vi "SNR_Analysis.vi"(5 "Ain (Input)":ext[](array[numeric])=array[16384 elements] format="%.2f", 7 "Input Ain Freq. (Hz)":dbl=10.0 format="%.4f", 8 "AC Analysis Parameters":T1={"DC Leakage"=5, "Number of Harmonics"=6, "HarmLeakage"=3, "FundLeakage"=15, "LoFreq (Hz)"=50.0, "HiFreq (Hz)"=100.0, "Window"=enum."None ", "Reference"=TRUE} {"HiFreq (Hz)" format="%.3g"; "LoFreq (Hz)" format="%.3g"; "FundLeakage" min=1 step=2; "HarmLeakage" min=1 step=2; "DC Leakage" min=1 step=1}, 9 "Ideal Sampling Rate":dbl=500.0 format="%.4f", 10 "Number of Bits":i8=24, 11 "Number of Samples":i32=16384) -> (0 "PSRR/CMRR/BW":T2={"Freq (Hz)"=[[0.0, 49.98779296875], [49.98779296875, 100.006103515625], [100.006103515625, 149.993896484375], [149.993896484375, 200.01220703125], [200.01220703125, 250.0], [0.0, 250.0], [49.98779296875, 100.006103515625]], "SNR (dBFS)"=[122.49294424672361, 122.35389846356063, 122.34393026582947, 122.45111299294416, 122.45121773152403, 115.43161378863995, 122.35389846356063], "Fund(dB)"=0.0} {"SNR (dBFS)" format="%.2f"; "Freq (Hz)" format="%.2f"}, 1 "FFT Magnitude Plot (dB)":cluster{i32, dbl, dbl[]}(graph)={0, 0.030517578125, array[8193 elements]}, 3 "ACParameter":T3)   [LabVIEW 2010]
uses:
  Controls/TYP_ACAnalysisParam.ctl
  <vilib>/Analysis/0measdsp.llb/Scaled Time Domain Window (DBL).vi
  <vilib>/Analysis/2dsp.llb/Real FFT.vi
  <vilib>/Analysis/4window.llb/General Cosine Window (DBL).vi
  <vilib>/Analysis/NI_AALPro.lvlib
  <vilib>/Analysis/NI_AALBase.lvlib
panel:
  in  "Case Constant\n(See Context Help) 2":bool=TRUE
  in  "Case Constant\n(See Context Help)":bool
  out "Fund (compensated)":ext=17592184028025.883722 format="%.2f"
  out "Freq (Hz)":dbl[][](array[numeric])=[[0.0, 49.98779296875], [49.98779296875, 100.006103515625], [100.006103515625, 149.993896484375], [149.993896484375, 200.01220703125], [200.01220703125, 250.0], [0.0, 250.0], [49.98779296875, 100.006103515625]] format="%.2f"
  out "SNR (dBFS)":dbl[](array[numeric])=[122.49294424672361, 122.35389846356063, 122.34393026582947, 122.45111299294416, 122.45121773152403, 115.43161378863995, 122.35389846356063] format="%.2f"
  out "CoherentGain":dbl=1.0
  out "EBW":dbl=1.0
  out "Window comp (dB)":dbl=-1.9937488104915246e-08
  out "Captured Data In Plot":ext[](graph)
  out "0dB Ref (Vrms^2)":ext=17592183947264.086
  out "0dB Ref (dB)":dbl=132.45319757443235
  out "Amplitude":dbl=8388607.5
  in  "BandMultiplier":ext=1.0 format="%#.2g"
  out "Noise Floor":ext[](array[numeric])=[9.9088974720743699205, 10.2312786546159955785, 10.254789094296063996, 10.0048011243385777027, 10.004559841966981927, 50.368426126531911098, 10.2312786546159955785] format="%_2f"
  out "Power Spec\n(No DC, Fund, Harmonics)":ext[](array[numeric]) format="%.2f"
  out "Numeric":i32=16
  out "Fund(dB)":dbl=132.45319759436984 format="%.2f"
  out "SNR 2":dbl=115.43161378863995 caption="SNR (dBFS)" format="%.2f"
  out "THD (dBc)":dbl=142.87642226580417 format="%.2f"
  out "Sum of Harms 2":ext=0.090714671632502579776 format="%.2f"
  out "SF":ext=132.453188236702958824 format="%.2f"
  out "WoSpur (dBFS)":ext=-145.06459832693680674 format="%.2f"
  out "Sum of Noise 2":ext=50.368426126531911098 format="%.2f"
  out "# of Harmonics (SNR)":u32=23
  out "debug waveform":ext[](graph)
  out "FFT":dbl[](graph)
  in  "Calculate (Actual)":bool
  out "Actual Ain Freq. (Hz)":ext=10.040283203125 format="%.6f"
  out "Low Code":i32=8388619
  out "High Code":i32=-8388612
  out "Performance Array":dbl[](array[numeric])=[115.43161378863995, 145.97359756076744, 154.47799816290882, 151.76114324149736, 115.39522693755671, 142.87642226580417, 148.72341540579788, 152.36692825715133, 18.876283544444636, 18.8823278718671, 8.453417793882701e-06] format="%.2f"
  out "Ampl.":dbl=8.453417793882701e-06 format="%.2f"
  out "3rdHarm@ Plot (dB)":dbl=-152.98466091578587 format="%.2f"
  out "2ndHarm @ Plot (dB)":dbl=-168.88785823900827 format="%.2f"
  out "1stHarm @ Plot (dB)":dbl=1.9937459683205816e-08 format="%.2f"
  out "5th HD":dbl=152.36692825715133 format="%.2f"
  out "4th HD":dbl=148.72341540579788 format="%.2f"
  out "Actual Sampling Rate":dbl=500.0 format="%.6f"
  out "Measured % of FS":dbl=100.00009732361634 format="%.2f"
  out "Actual Number of Codes":u32=16777216
  out "min Code":i32
  out "max Code":i32=16777215
  out "enob":dbl=18.8823278718671 format="%.2f"
  out "ENOB":dbl=18.876283544444636 format="%.2f"
  out "3rd HD":dbl=151.76114324149736 format="%.2f"
  out "2nd HD (dBc)":dbl=154.47799816290882 format="%.2f"
  out "SFDR (dBc)":dbl=145.97359756076744 format="%.2f"
  out "THD (dBc)":dbl=136.05208345742915 format="%.2f"
  out "SNR":dbl=115.43272182505751 caption="SNR (dBc)" format="%.2f"
  out "SNRD":dbl=115.39522693755671 caption="SNRD (dBFS)" format="%.2f"
  out "max Harmonic":ext=0.044459032074172995111 format="%.2f"
  out "Fund":ext=17592184028025.883722 format="%.2f"
  out "Harmonic Spectrum":ext[](array[numeric])=[0.006273645043968196789, 0.011727499829014819744, 0.023603598512384399172, 0.010200628560604323592, 0.010739693568795177, 0.028169606117735663479, 0.022250863209773356736, 0.024737167818243943097, 0.029718462590962836569, 0.018866757624148633877, 0.01857286143792718754, 0.012624382823140385245, 0.0088173049746291707555, 0.0150888701235834066326, 0.03351059535541610953, 0.010733796961532902247, 0.044459032074172995111, 0.024528219551121035937, 0.005135965514516267305, 0.0023413793635542205077, 0.012309499745878399, 0.041509770726511618748, 0.020708228636082309619] format="%.2f"
  out "Sum of Noise":ext=50.355577026708861234 format="%.2f"
  out "Sum of Harms":ext=0.436627830163697358 format="%.2f"
  out "Bin Locations":i32[](array[numeric])
  out "Tone Bin#":u32=329
  out "Nyquist":i32=8192
  out "FFT Power Spectrum":ext[](array[numeric]) format="%.2f"
  out "Amplitude Compensation":ext=0.9999980535305147 format="%.6f"
  out "Half of Codes":ext=8388608.0 format="%.2f"
  out "Ain":ext[](array[numeric]) format="%.2f"
  # "AC Analysis"
  # "Fs"
  # "Fin"
  # "dBFS"
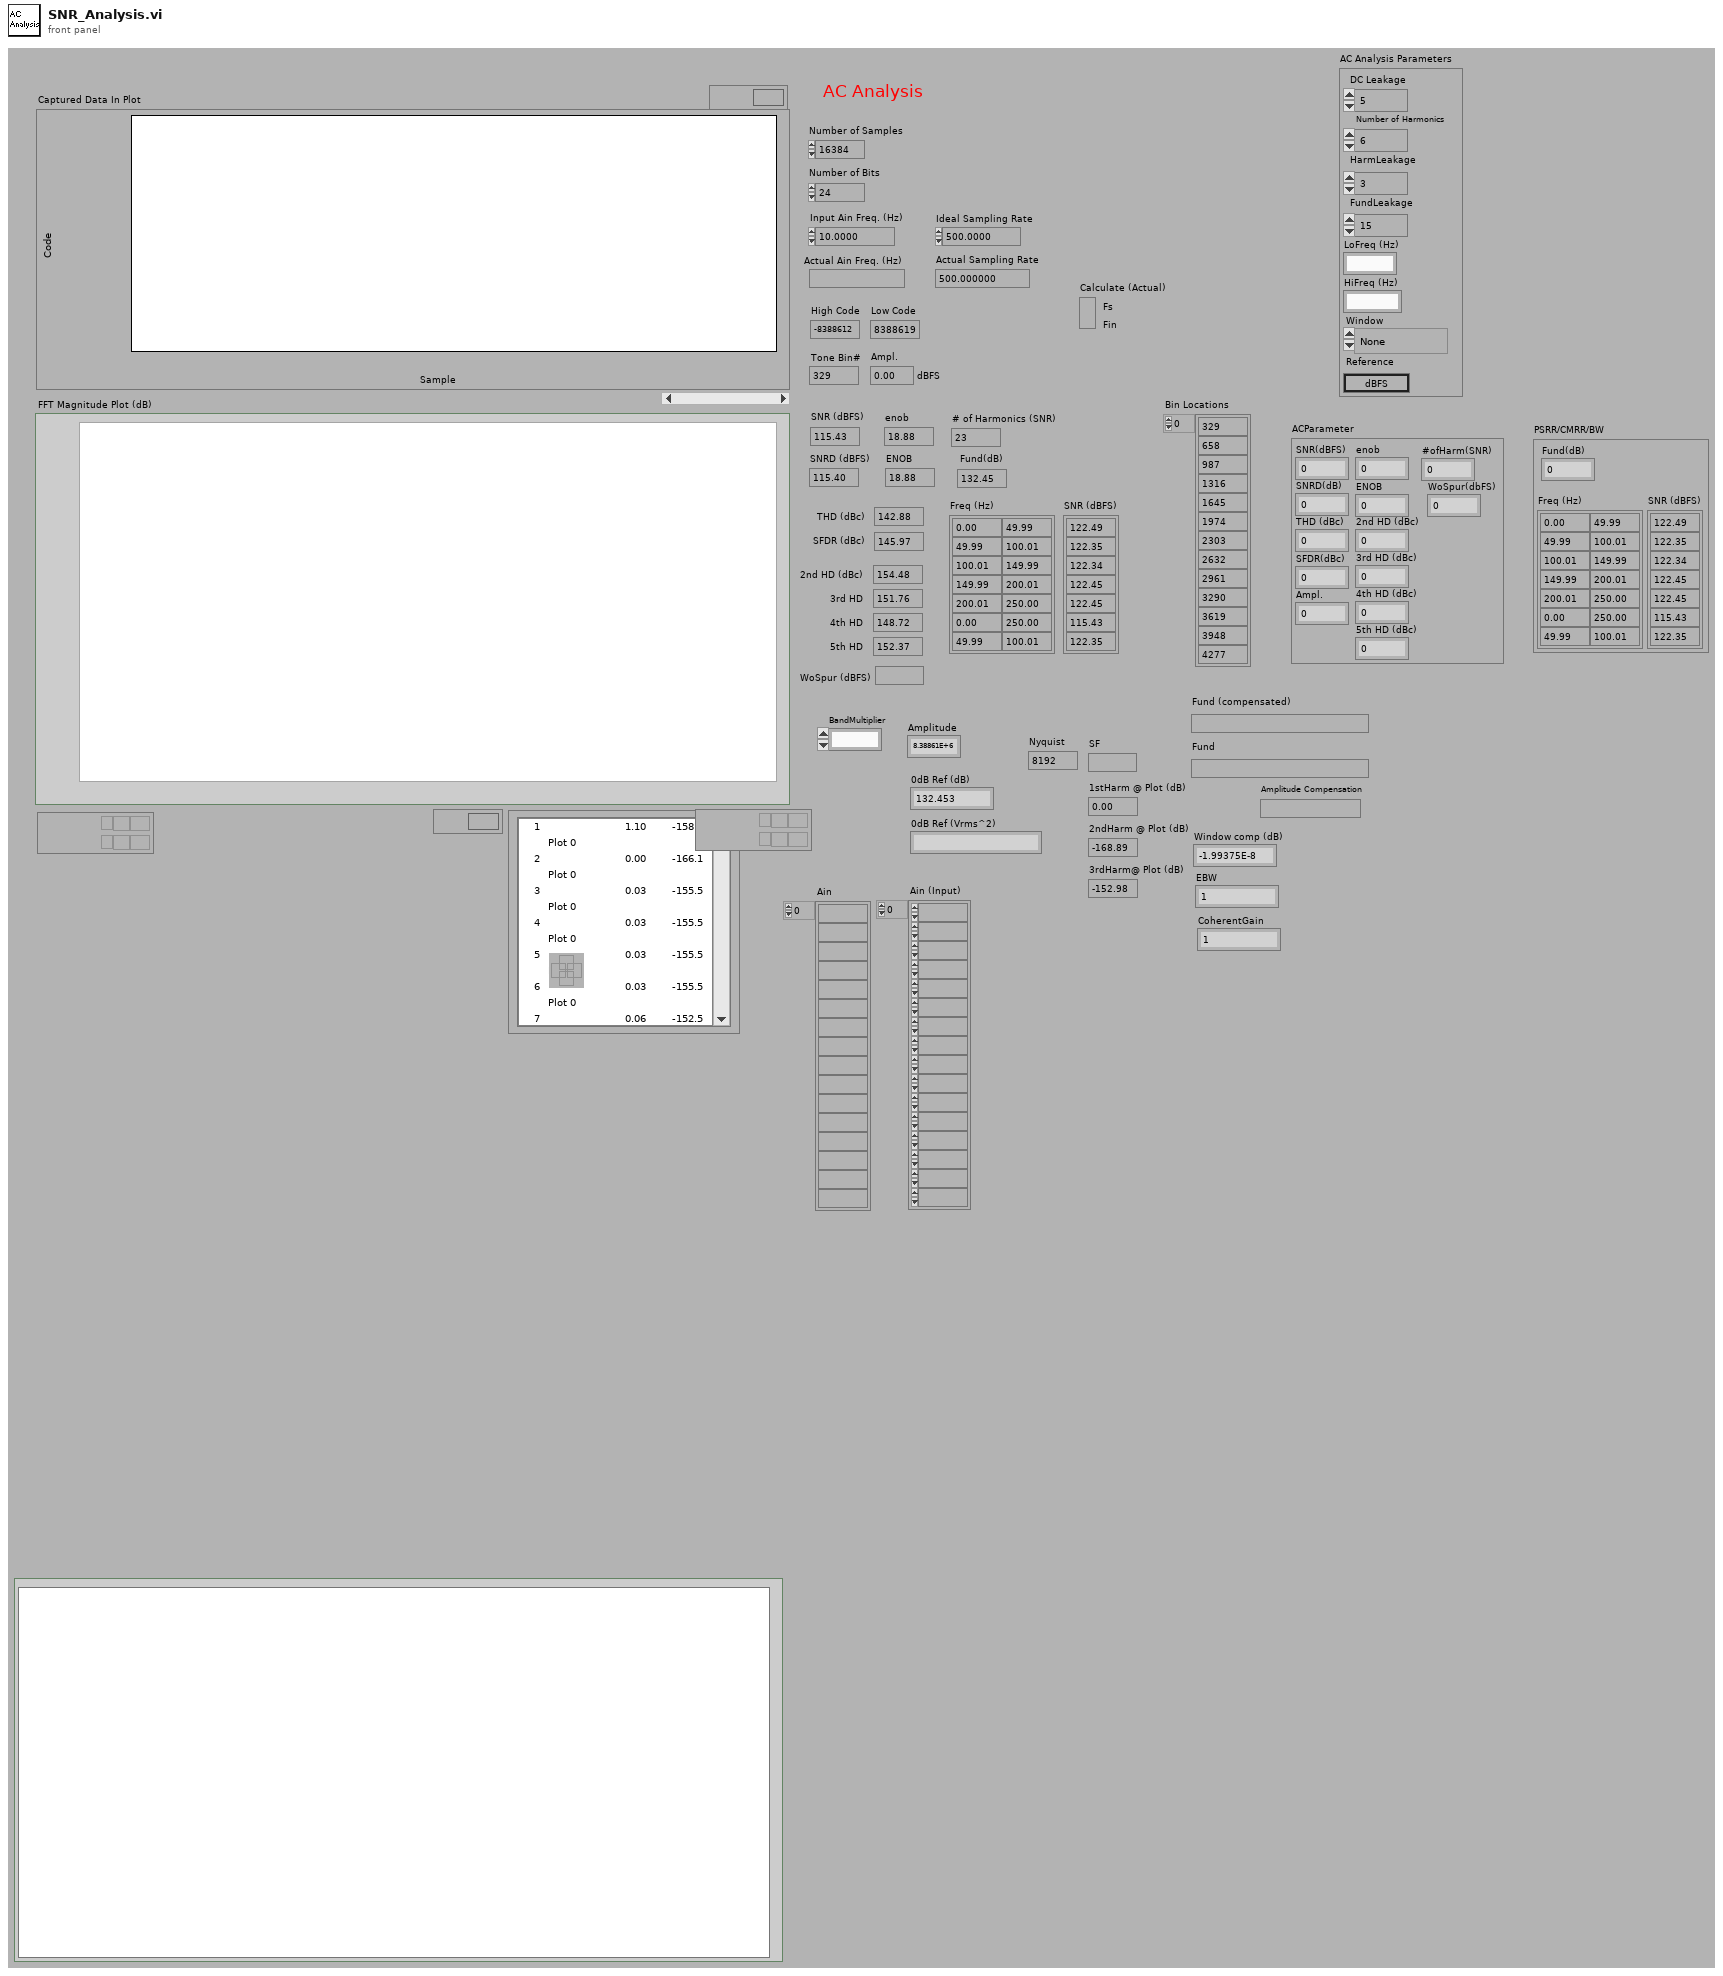
[diagram p1: front panel]
types:
  T1 = typedef "TYP_ACAnalysisParam.ctl" = cluster{"DC Leakage":i8, "Number of Harmonics":i8, "HarmLeakage":i8, "FundLeakage":i32, "LoFreq (Hz)":ext, "HiFreq (Hz)":ext, "Window":enum16{"None ", "Hanning", "Hamming", "Blackman-Harris", "Exact Blackman", "Blackman", "Flat Top", "4 Term B-Harris ", "7 Term B-Harris", "Low Sidelobe"}, "Reference":bool}
  T2 = cluster{"Freq (Hz)":dbl[][], "SNR (dBFS)":dbl[], "Fund(dB)":dbl}
  T3 = cluster{"SNR(dBFS)":dbl, "SNRD(dB)":dbl, "THD (dBc)":dbl, "SFDR(dBc)":dbl, "ENOB":dbl, "enob":dbl, "#ofHarm(SNR)":dbl, "WoSpur(dbFS)":dbl, "2nd HD (dBc)":dbl, "3rd HD (dBc)":dbl, "4th HD (dBc)":dbl, "5th HD (dBc)":dbl, "Ampl.":dbl}
  T4 = enum16{"None ", "Hanning", "Hamming", "Blackman-Harris", "Exact Blackman", "Blackman", "Flat Top", "4 Term B-Harris ", "7 Term B-Harris", "Low Sidelobe"}
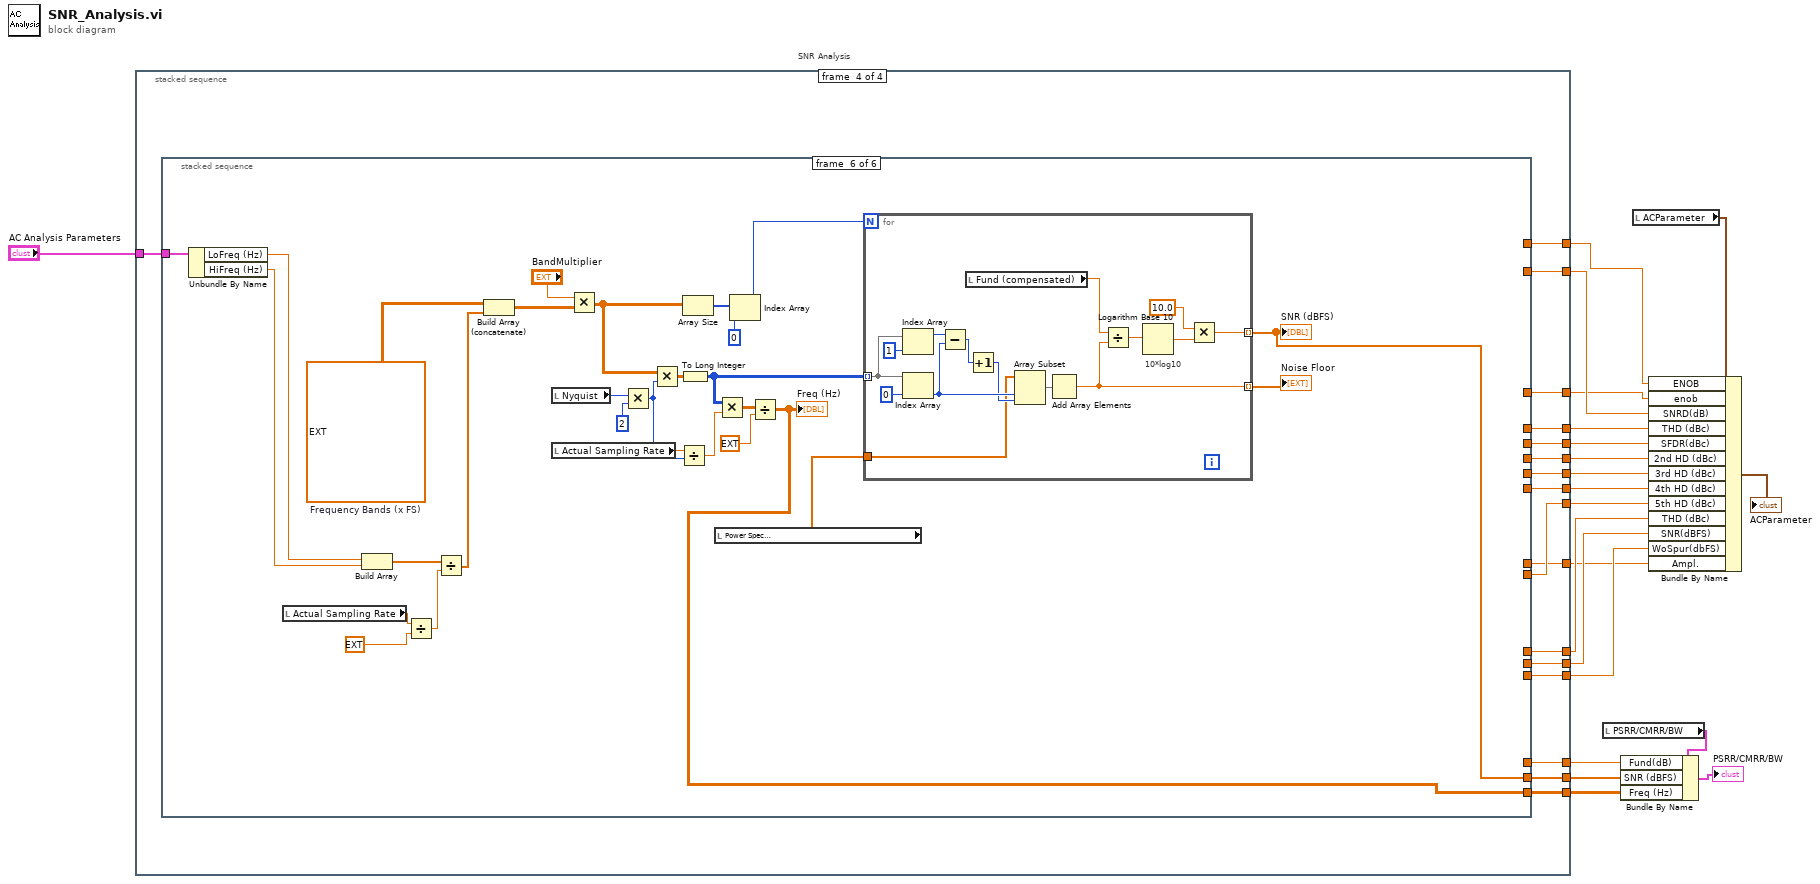
[diagram p0: block diagram]
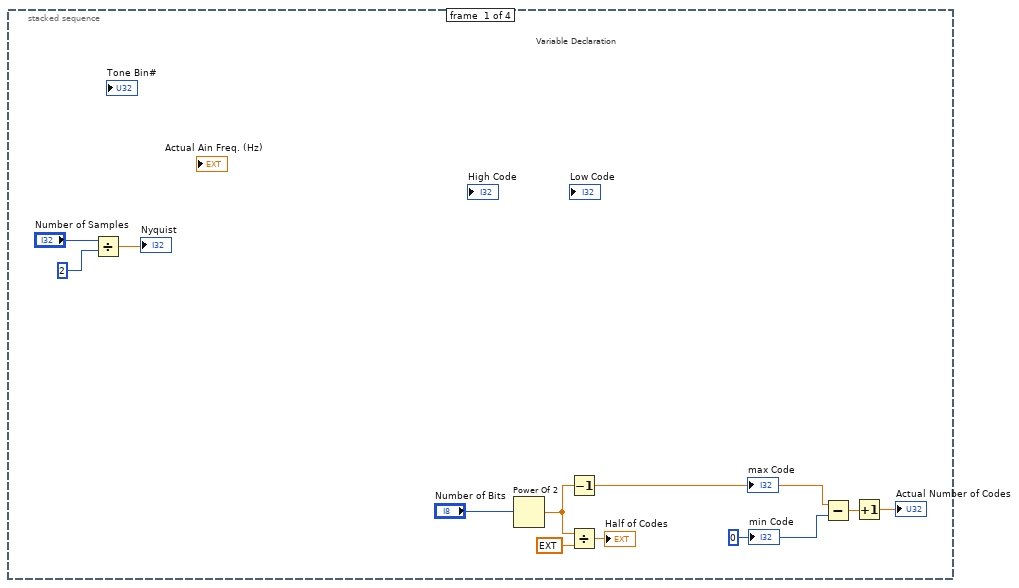
[diagram p2: hidden frame]
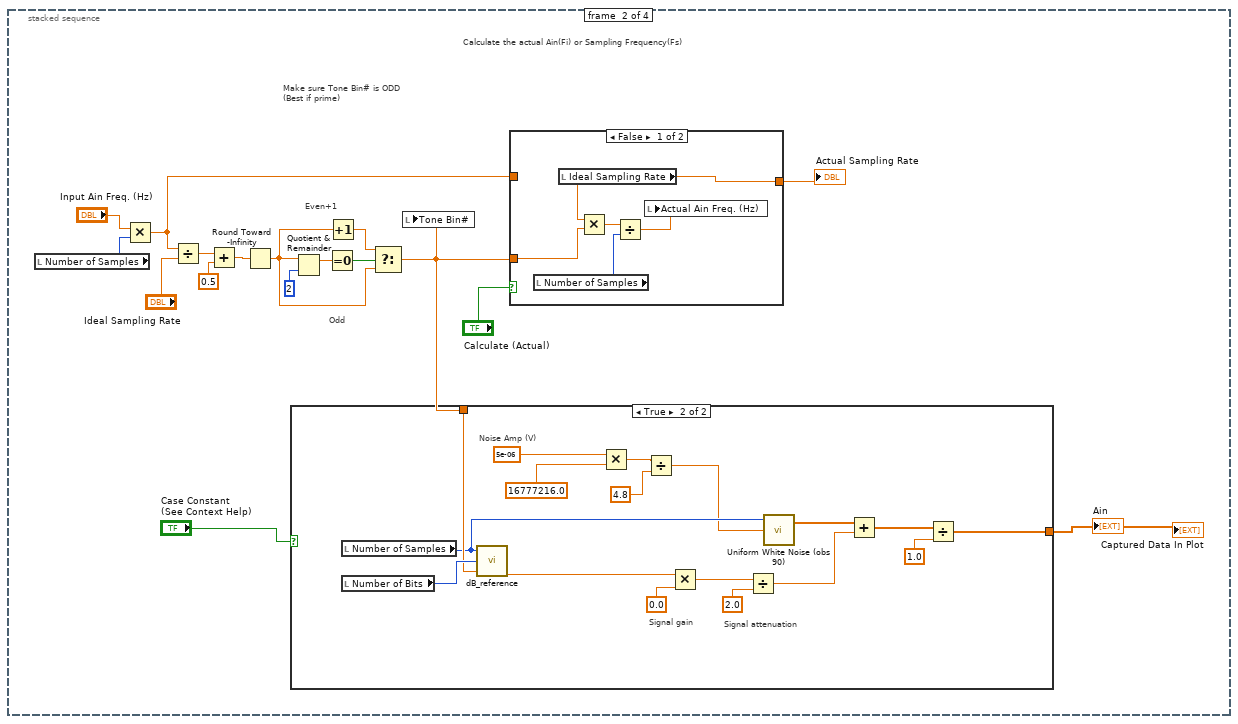
[diagram p3: hidden frame]
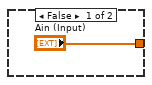
[diagram p4: hidden frame]
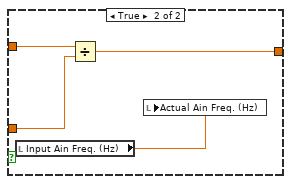
[diagram p5: hidden frame]
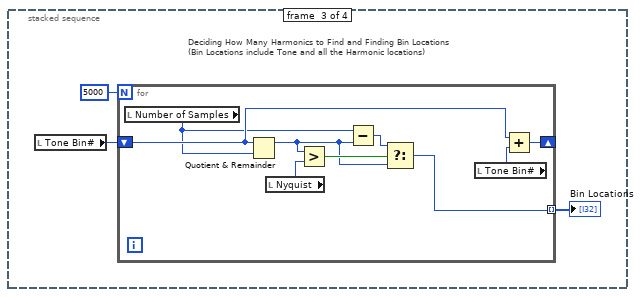
[diagram p6: hidden frame]
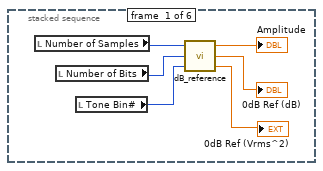
[diagram p7: hidden frame]
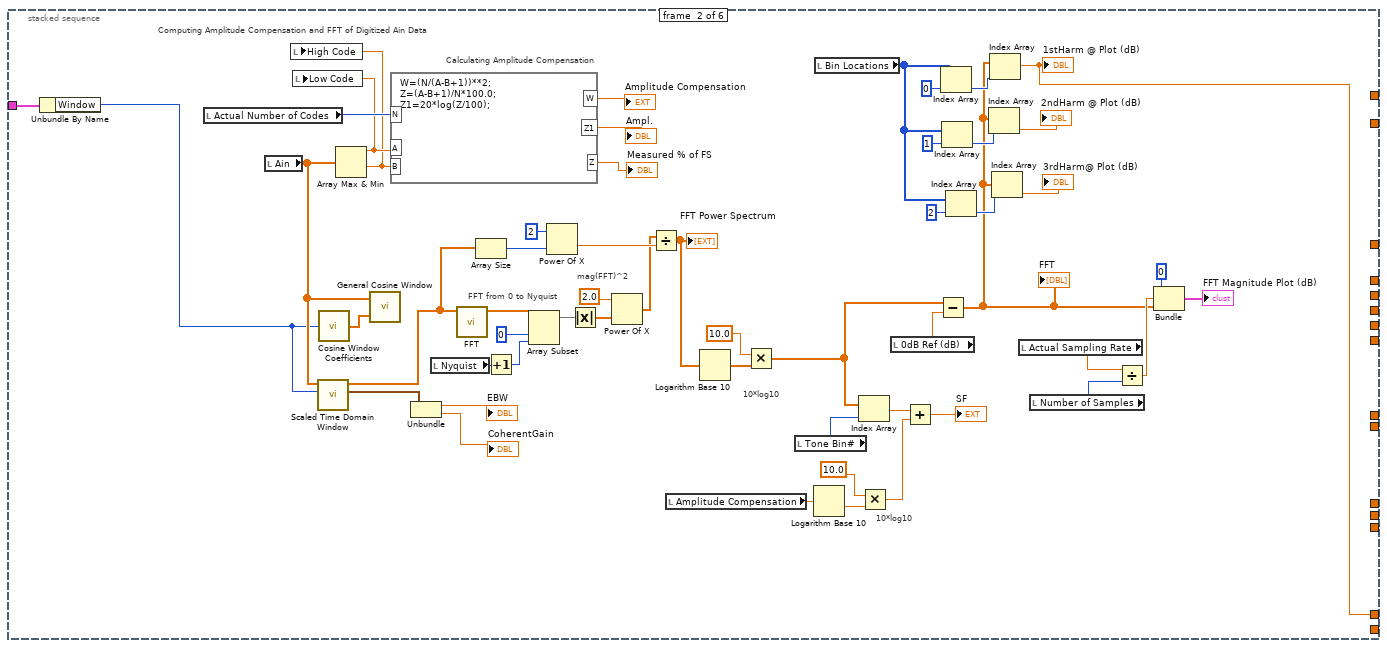
[diagram p8: hidden frame]
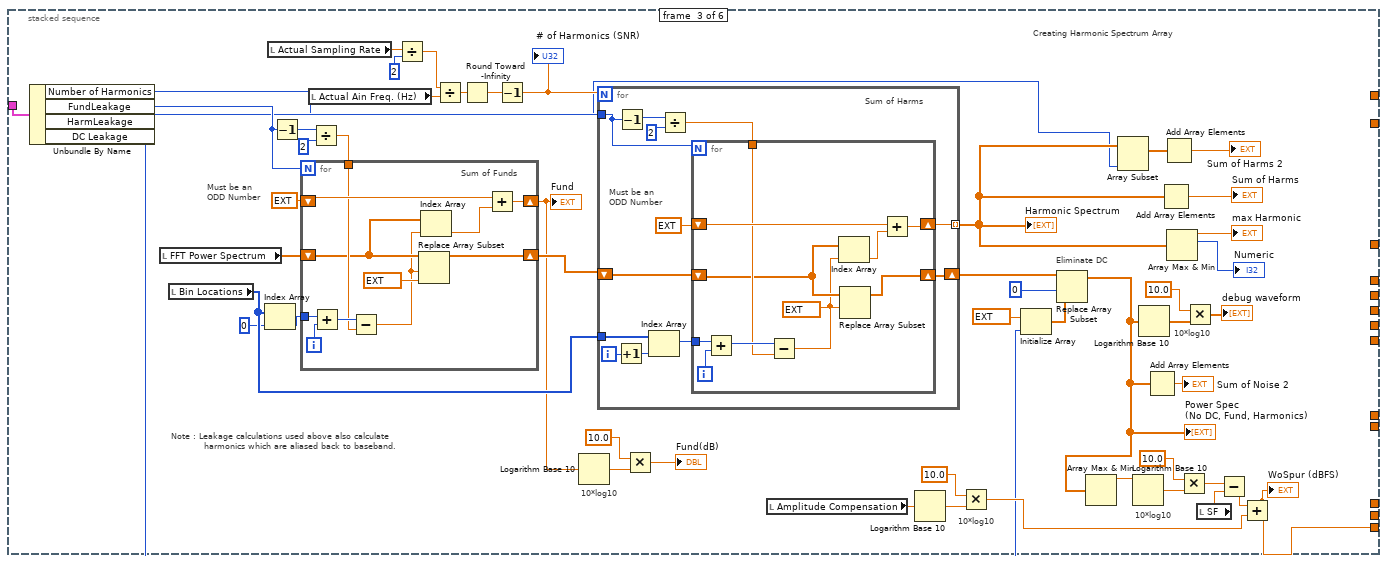
[diagram p9: hidden frame]
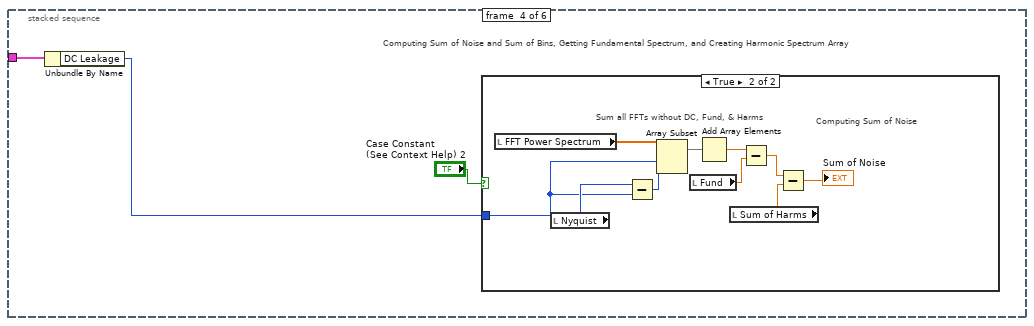
[diagram p10: hidden frame]
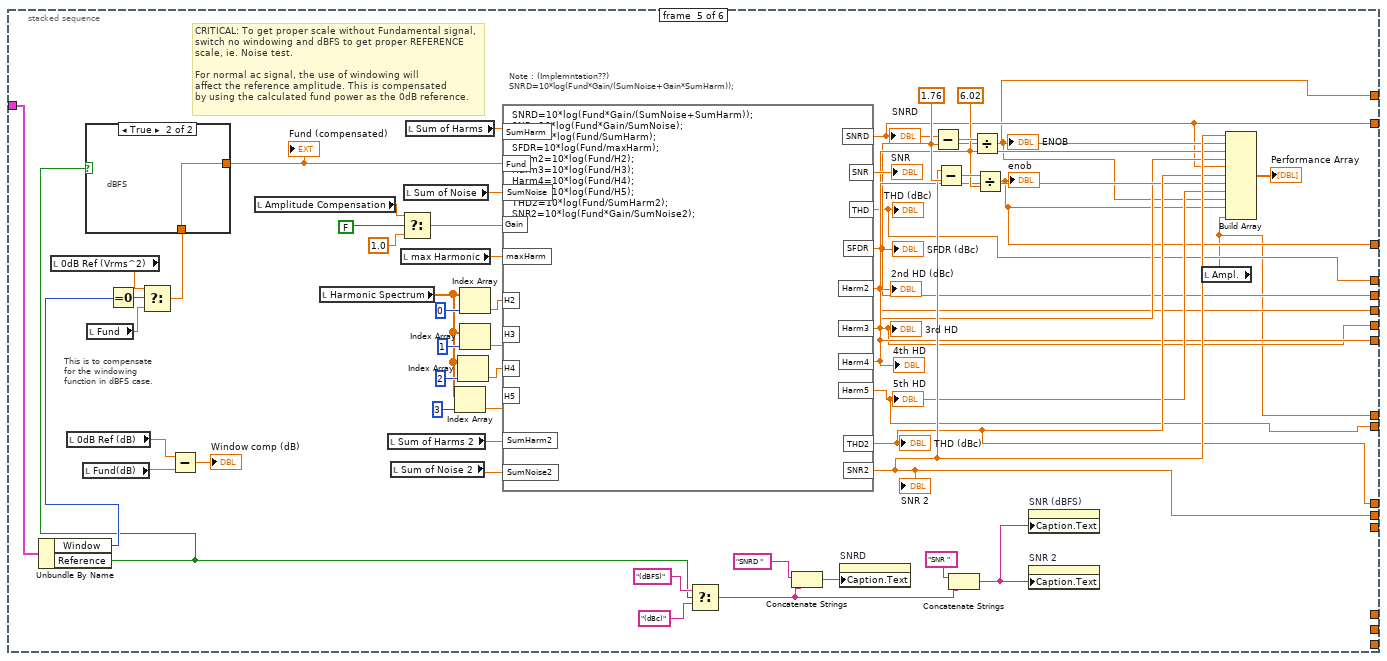
[diagram p12: hidden frame]
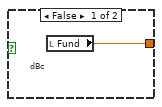
[diagram p13: hidden frame]
diagram:
  # "SNR Analysis"
  n1 = stacked-sequence {
    tunnel: [_ _ _ w105] -> w17
    tunnel: [_ _ _ w104] -> w16
    tunnel: [_ _ _ w103] -> w15
    tunnel: [_ _ _ w102] -> w14
    tunnel: [_ _ _ w101] -> w13
    tunnel: [_ _ _ w100] -> w12
    tunnel: [_ _ _ w99] -> w11
    tunnel: [_ _ _ w98] -> w10
    tunnel: [_ _ _ w97] -> w9
    tunnel: [_ _ _ w96] -> w8
    tunnel: [_ _ _ w95] -> w7
    tunnel: [_ _ _ w94] -> w6
    tunnel: [_ _ _ w93] -> w5
    tunnel: [_ _ _ w92] -> w4
    tunnel: [_ _ _ w91] -> w3
    tunnel: [_ _ _ w90] -> w2
    tunnel: "AC Analysis Parameters" -> [_ _ _ w89]
    frame #0 {
      w26 = 0 ("min Code")
      # "Variable Declaration"
      n2 = Divide(x="Number of Samples", y=2) -> (x/y=→"Nyquist":dbl)
      n3 = Power Of 2(x="Number of Bits") -> (2^x=w23:dbl)
      n4 = Decrement(x=w23) -> (x-1=w22:dbl)
      "max Code" <- w22
      n5 = Divide(x=w23, y=ext 2.0) -> (x/y=→"Half of Codes":ext)
      n6 = Subtract(x=w22, y=w26) -> (x-y=w25:dbl)
      n7 = Increment(x=w25) -> (x+1=→"Actual Number of Codes":dbl)
      "min Code" <- w26
    }
    frame #1 {
      # "Calculate the actual Ain(Fi) or Sampling Frequency(Fs)"
      # "Make sure Tone Bin# is ODD\n(Best if prime)"
      # "Even+1"
      # "Odd"
      n8 = local read "Number of Samples"() -> (w42:i32)
      n9 = Multiply(x="Input Ain Freq. (Hz)", y=w42) -> (x*y=w38:dbl)
      n10 = Divide(x=w38, y="Ideal Sampling Rate") -> (x/y=w40:dbl)
      n11 = Add(x=w40, y=0.5) -> (x+y=w39:dbl)
      n12 = Round Toward -Infinity(1:w39) -> (0:w48:dbl)
      n13 = Quotient & Remainder(x=w48, y=2) -> (x-y*floor(x/y)=w45:dbl)  [unwired: 1 out]
      n14 = Equal To 0?(x=w45) -> (x = 0?=w46:bool)
      n15 = Increment(x=w48) -> (x+1=w47:dbl)
      n16 = Select(t=w47, s=w46, f=w48) -> (s? t:f=w35:dbl)
      n17 = case shown="True" "Case Constant\n(See Context Help)" {
        tunnel: w35 -> [_ w65]
        tunnel: ["Ain (Input)" w51] -> w33
        frame False {
        }
        frame True {
          # "Signal attenuation"
          # "Signal gain"
          # "Noise Amp (V)"
          n18 = local read "Number of Samples"() -> (w64:i32)
          n19 = local read "Number of Bits"() -> (w67:i8)
          n20 = call "dB_reference.vi"("Tone Bin#"=w65, "Number of Bits"=w67, "Number of Samples"=w64) -> ("0dB Ref (Vrms^2)"=w55:ext)  [unwired: 2 out]
          n21 = Multiply(x=5e-06 ("y"), y=16777216.0) -> (x*y=w62:dbl)
          n22 = Divide(x=w62, y=4.8) -> (x/y=w61:dbl)
          n23 = Multiply(x=w55, y=0.0) -> (x*y=w54:ext)
          n24 = Divide(x=w54, y=2.0) -> (x/y=w53:ext)
          n25 = call <vilib>:"Uniform White Noise (obs 90).vi"("amplitude"=w61, "samples"=w64) -> ("uniform white noise"=w58:dbl[])  [unwired: 1 in, 1 out]
          n26 = Add(x=w58, y=w53) -> (x+y=w57:ext[])
          n27 = Divide(x=w57, y=1.0) -> (x/y=w51:ext[])
        }
      }
      "Captured Data In Plot" <- w33
      "Ain" <- w33
      n28 = local write "Tone Bin#"(w35) -> ()
      n29 = case shown="False" "Calculate (Actual)" {
        tunnel: w38 -> [_ w76]
        tunnel: w35 -> [w72 w75]
        tunnel: [w68 w74] -> w37
        frame False {
          n30 = local read "Number of Samples"() -> (w70:i32)
          n31 = local read "Ideal Sampling Rate"() -> (w68:dbl)
          n32 = Multiply(x=w68, y=w72) -> (x*y=w71:dbl)
          n33 = Divide(x=w71, y=w70) -> (x/y=w69:dbl)
          n34 = local write "Actual Ain Freq. (Hz)"(w69) -> ()
        }
        frame True {
          n35 = local read "Input Ain Freq. (Hz)"() -> (w73:dbl)
          n36 = Divide(x=w76, y=w75) -> (x/y=w74:dbl)
          n37 = local write "Actual Ain Freq. (Hz)"(w73) -> ()
        }
      }
      "Actual Sampling Rate" <- w37
    }
    frame #2 {
      # "Deciding How Many Harmonics to Find and Finding Bin Locations\n(Bin Locations include Tone and all the Harmonic locations)"
      n38 = local read "Tone Bin#"() -> (w78:u32)
      n39 = for {
        N: 5000 -> [_]
        shift-right: [w87] -> _
        shift-left: w78 -> [w86]
        tunnel: [w80] -> w77 mode=indexing
        n40 = local read "Number of Samples"() -> (w83:i32)
        n41 = Quotient & Remainder(x=w86, y=w83) -> (x-y*floor(x/y)=w81:u32)  [unwired: 1 out]
        n42 = local read "Nyquist"() -> (w88:i32)
        n43 = Greater?(x=w81, y=w88) -> (0:w84:bool)
        n44 = Subtract(x=w83, y=w81) -> (x-y=w82:u32)
        n45 = Select(t=w82, s=w84, f=w81) -> (s? t:f=w80:u32)
        n46 = local read "Tone Bin#"() -> (w85:u32)
        n47 = Add(x=w86, y=w85) -> (x+y=w87:u32)
      }
      "Bin Locations" <- w77
    }
    frame #3 {
      n48 = stacked-sequence {
        tunnel: [_ _ w171 _ _ _] -> w105
        tunnel: [_ w114 _ _ _ _] -> w104
        tunnel: [_ _ _ _ w277 _] -> w103
        tunnel: [_ _ _ _ w276 _] -> w102
        tunnel: [_ _ _ _ w275 _] -> w101
        tunnel: [_ _ _ _ w274 _] -> w100
        tunnel: [_ _ _ _ w273 _] -> w99
        tunnel: [_ _ _ _ w272 _] -> w98
        tunnel: [_ _ _ _ w271 _] -> w97
        tunnel: [_ _ _ _ w270 _] -> w96
        tunnel: [_ _ _ _ w269 _] -> w95
        tunnel: [_ _ _ _ w268 _] -> w94
        tunnel: [_ _ _ _ w267 _] -> w93
        tunnel: [_ _ _ _ w266 _] -> w92
        tunnel: [_ _ _ _ _ w323] -> w91
        tunnel: [_ _ _ _ _ w322] -> w90
        tunnel: w89 -> [_ w113 w169 w251 w265 w321]
        frame #0 {
          n49 = local read "Number of Samples"() -> (w111:i32)
          n50 = local read "Number of Bits"() -> (w110:i8)
          n51 = local read "Tone Bin#"() -> (w109:u32)
          n52 = call "dB_reference.vi"("Tone Bin#"=w109, "Number of Bits"=w110, "Number of Samples"=w111) -> ("0dB Ref (Vrms^2)"=→"0dB Ref (Vrms^2)":ext, "0dB Ref (dB)"=→"0dB Ref (dB)":dbl, "Amplitude"=→"Amplitude":dbl)
        }
        frame #1 {
          # "10*log10"
          # "FFT from 0 to Nyquist"
          # "10*log10"
          # "Computing Amplitude Compensation and FFT of Digitized Ain Data"
          # "Calculating Amplitude Compensation"
          # "mag(FFT)^2"
          n53 = Unbundle By Name(w113) -> ("Window"=w112:T4)
          n54 = local read "Actual Number of Codes"() -> (w164:u32)
          n55 = local read "Ain"() -> (w125:ext[])
          n56 = call-poly <vilib>:"Scaled Time Domain Window.vi"("window"=w112, "X"=w125) -> ("window properties"=w123:cluster{"eq noise BW":dbl, "coherent gain":dbl}, "Windowed X"=w124:dbl[])  [unwired: 1 in, 7 out]
          n57 = call <vilib>:"Cosine Window Coefficients.vi"("window"=w112) -> ("WinCoefficients"=w129:dbl[])
          n58 = Array Max & Min(array=w125) -> (max value=w142:ext, min value=w141:ext)  [unwired: 2 out]
          n59 = local write "High Code"(w141) -> ()
          n60 = local write "Low Code"(w142) -> ()
          n61 = call-poly <vilib>:"General Cosine Window.vi"("Cosine Coefficients"=w129, "X"=w125) -> ()  [unwired: 2 out]
          n62 = formula code="W=(N/(A-B+1))**2;\nZ=(A-B+1)/N*100.0;\nZ1=20*log(Z/100);"("A"=w142, "B"=w141, "N"=w164) -> ("W"=→"Amplitude Compensation":dbl, "Z"=→"Measured % of FS":dbl, "Z1"=→"Ampl.":dbl)
          n63 = Unbundle(w123) -> ("eq noise BW"=→"EBW":dbl, "coherent gain"=→"CoherentGain":dbl)
          n64 = local read "Nyquist"() -> (w158:i32)
          n65 = call-poly <vilib>:"FFT.vi"("X"=w124) -> ("FFT {X}"=w154:cdb[])  [unwired: 2 in, 8 out]
          n66 = Array Size(array=w124) -> (size(s)=w134:i32)
          n67 = Increment(x=w158) -> (x+1=w157:i32)
          n68 = Array Subset(array=w154, index=0, length=w157) -> (w156:cdb[])
          n69 = Power Of X(1:w134, 2:2 ("y")) -> (0:w132:dbl)
          n70 = Absolute Value(x=w156) -> (abs(x)=w162:dbl[])
          n71 = Power Of X(1:w162, 2:2.0) -> (0:w131:dbl[])
          n72 = Divide(x=w131, y=w132) -> (x/y=w130:dbl[])
          "FFT Power Spectrum" <- w130
          n73 = local read "Amplitude Compensation"() -> (w136:ext)
          n74 = Logarithm Base 10(1:w130) -> (0:w160:dbl[])
          n75 = Multiply(x=10.0, y=w160) -> (x*y=w128:dbl[])
          n76 = local read "Tone Bin#"() -> (w140:u32)
          n77 = Logarithm Base 10(1:w136) -> (0:w137:ext)
          n78 = local read "Bin Locations"() -> (w148:i32[])
          n79 = Index Array(array=w128, index=w140) -> (element=w139:dbl)
          n80 = Multiply(x=10.0, y=w137) -> (x*y=w135:ext)
          n81 = local read "0dB Ref (dB)"() -> (w127:dbl)
          n82 = Add(x=w139, y=w135) -> (x+y=→"SF":ext)
          n83 = Subtract(x=w128, y=w127) -> (x-y=w115:dbl[])
          "FFT" <- w115
          n84 = Index Array(array=w148, index=0 ("Index")) -> (element=w151:i32)
          n85 = Index Array(array=w148, index=1 ("Index")) -> (element=w150:i32)
          n86 = Index Array(array=w148, index=2 ("Index")) -> (element=w149:i32)
          n87 = Index Array(array=w115, index=w150) -> (element=→"2ndHarm @ Plot (dB)":dbl)
          n88 = Index Array(array=w115, index=w151) -> (element=w114:dbl)
          "1stHarm @ Plot (dB)" <- w114
          n89 = Index Array(array=w115, index=w149) -> (element=→"3rdHarm@ Plot (dB)":dbl)
          n90 = local read "Actual Sampling Rate"() -> (w120:dbl)
          n91 = local read "Number of Samples"() -> (w119:i32)
          n92 = Divide(x=w120, y=w119) -> (x/y=w118:dbl)
          n93 = Bundle(0, w118, w115) -> (→"FFT Magnitude Plot (dB)":cluster{i32, dbl, dbl[]})  [unwired: 1 out]
        }
        frame #2 {
          # "10*log10"
          # "10*log10"
          # "Eliminate DC"
          # "10*log10"
          # "10*log10"
          # "Creating Harmonic Spectrum Array"
          # "Must be an\nODD Number"
          # "Note : Leakage calculations used above also calculate\n           harmonics which are aliased back to baseband."
          n94 = Unbundle By Name(w169) -> ("Number of Harmonics"=w165:i8, "FundLeakage"=w168:i32, "HarmLeakage"=w167:i8, "DC Leakage"=w166:i8)
          n95 = local read "FFT Power Spectrum"() -> (w182:ext[])
          n96 = local read "Bin Locations"() -> (w215:i32[])
          n97 = Index Array(array=w215, index=0 ("Index")) -> (element=w211:i32)
          n98 = local read "Actual Sampling Rate"() -> (w200:dbl)
          n99 = Decrement(x=w168) -> (x-1=w212:i32)
          n100 = local read "Actual Ain Freq. (Hz)"() -> (w203:ext)
          n101 = Divide(x=w212, y=2) -> (x/y=w214:dbl)
          n102 = for {
            N: w168 -> [_]
            shift-right: [w222] -> w185
            shift-left: ext 0.0 -> [w223]
            tunnel: w211 -> [w224]
            tunnel: w214 -> [w221]
            shift-right: [w217] -> w208
            shift-left: w182 -> [w218]
            i -> [w226]
            # "Sum of Funds"
            n103 = Add(x=w224, y=w226) -> (x+y=w225:i32)
            n104 = Subtract(x=w225, y=w221) -> (x-y=w216:dbl)
            n105 = Replace Array Subset(array=w218, new element=ext 0.0 ("Element Data"), index=w216) -> (w217:ext[])
            n106 = Index Array(array=w218, index=w216) -> (element=w220:ext)
            n107 = Add(x=w223, y=w220) -> (x+y=w222:ext)
          }
          "Fund" <- w185
          n108 = Divide(x=w200, y=2) -> (x/y=w204:dbl)
          n109 = Divide(x=w204, y=w203) -> (x/y=w202:ext)
          n110 = Round Toward -Infinity(1:w202) -> (0:w199:ext)
          n111 = Decrement(x=w199) -> (x-1=w191:ext)
          "# of Harmonics (SNR)" <- w191
          n112 = Logarithm Base 10(1:w185) -> (0:w187:ext)
          n113 = for {
            N: w191 -> [_]
            tunnel: [w236] -> w183 mode=indexing
            tunnel: w215 -> [w230]
            shift-right: [w228] -> w172
            shift-left: w208 -> [w229]
            tunnel: w167 -> [w227]
            i -> [w238]
            # "Must be an\nODD Number"
            # "Sum of Harms"
            n114 = Increment(x=w238) -> (x+1=w237:i32)
            n115 = Decrement(x=w227) -> (x-1=w234:i8)
            n116 = Index Array(array=w230, index=w237) -> (element=w231:i32)
            n117 = Divide(x=w234, y=2) -> (x/y=w233:dbl)
            n118 = for {
              N: w227 -> [_]
              shift-right: [w245] -> w236
              shift-left: ext 0.0 -> [w248]
              tunnel: w233 -> [w246]
              tunnel: w231 -> [w244]
              shift-right: [w240] -> w228
              shift-left: w229 -> [w241]
              i -> [w249]
              n119 = Add(x=w244, y=w249) -> (x+y=w247:i32)
              n120 = Subtract(x=w247, y=w246) -> (x-y=w239:dbl)
              n121 = Index Array(array=w241, index=w239) -> (element=w243:ext)
              n122 = Replace Array Subset(array=w241, new element=ext 0.0001 ("Element Data"), index=w239) -> (w240:ext[])
              n123 = Add(x=w248, y=w243) -> (x+y=w245:ext)
            }
          }
          "Harmonic Spectrum" <- w183
          n124 = Multiply(x=10.0, y=w187) -> (x*y=→"Fund(dB)":ext)
          n125 = local read "Amplitude Compensation"() -> (w181:ext)
          n126 = Logarithm Base 10(1:w181) -> (0:w180:ext)
          n127 = Multiply(x=10.0, y=w180) -> (x*y=w177:ext)
          n128 = Initialize Array(ext 1e-15 ("Element Data"), w166) -> (w173:ext[])
          n129 = Replace Array Subset(array=w172, new element=w173, index=0) -> (w176:ext[])
          "Power Spec\n(No DC, Fund, Harmonics)" <- w176
          n130 = Array Max & Min(array=w176) -> (max value=w196:ext)  [unwired: 3 out]
          n131 = Array Subset(array=w183, length=w165) -> (w192:ext[])  [unwired: 1 in]
          n132 = Logarithm Base 10(1:w196) -> (0:w195:ext)
          n133 = Logarithm Base 10(1:w176) -> (0:w207:ext[])
          n134 = Add Array Elements(numeric array=w176) -> (sum=→"Sum of Noise 2":ext)
          n135 = Add Array Elements(numeric array=w183) -> (sum=→"Sum of Harms":ext)
          n136 = Add Array Elements(numeric array=w192) -> (sum=→"Sum of Harms 2":ext)
          n137 = Array Max & Min(array=w183) -> (max value=→"max Harmonic":ext, max index (indices)=→"Numeric":i32)  [unwired: 2 out]
          n138 = Multiply(x=10.0, y=w195) -> (x*y=w197:ext)
          n139 = Multiply(x=10.0, y=w207) -> (x*y=→"debug waveform":ext[])
          n140 = local read "SF"() -> (w198:ext)
          n141 = Subtract(x=w197, y=w198) -> (x-y=w178:ext)
          n142 = Add(x=w178, y=w177) -> (x+y=w171:ext)
          "WoSpur (dBFS)" <- w171
        }
        frame #3 {
          # "Computing Sum of Noise and Sum of Bins, Getting Fundamental Spectrum, and Creating Harmonic Spectrum Array"
          n143 = Unbundle By Name(w251) -> ("DC Leakage"=w250:i8)
          n144 = case shown="True" "Case Constant\n(See Context Help) 2" {
            tunnel: w250 -> [_ w253]
            frame False {
            }
            frame True {
              # "Sum all FFTs without DC, Fund, & Harms"
              # "Computing Sum of Noise"
              n145 = local read "FFT Power Spectrum"() -> (w257:ext[])
              n146 = local read "Nyquist"() -> (w255:i32)
              n147 = Subtract(x=w255, y=w253) -> (x-y=w256:i32)
              n148 = Array Subset(array=w257, index=w253, length=w256) -> (w262:ext[])
              n149 = local read "Fund"() -> (w259:ext)
              n150 = Add Array Elements(numeric array=w262) -> (sum=w261:ext)
              n151 = local read "Sum of Harms"() -> (w258:ext)
              n152 = Subtract(x=w261, y=w259) -> (x-y=w260:ext)
              n153 = Subtract(x=w260, y=w258) -> (x-y=→"Sum of Noise":ext)
            }
          }
        }
        frame #4 {
          w307 = 6.02
          w310 = 1.76
          # "This is to compensate\nfor the windowing \nfunction in dBFS case."
          # "CRITICAL: To get proper scale without Fundamental signal, \nswitch no windowing and dBFS to get proper REFERENCE\nscale, ie. Noise test.\n\nFor normal ac signal, the use of windowing will\naffect the reference amplitude. This is compensated \nby using the calculated fund power as the 0dB reference."
          # "Note : (Implemntation??)\nSNRD=10*log(Fund*Gain/(SumNoise+Gain*SumHarm));"
          n154 = Unbundle By Name(w265) -> ("Window"=w264:T4, "Reference"=w263:bool)
          n155 = local read "0dB Ref (Vrms^2)"() -> (w288:ext)
          n156 = local read "0dB Ref (dB)"() -> (w292:dbl)
          n157 = local read "Fund(dB)"() -> (w290:dbl)
          n158 = local read "Fund"() -> (w287:ext)
          n159 = Equal To 0?(x=w264) -> (x = 0?=w289:bool)
          n160 = Select(t=w288, s=w289, f=w287) -> (s? t:f=w286:ext)
          n161 = case shown="True" w263 {
            tunnel: [w317 w318] -> w285
            tunnel: w286 -> [_ w318]
            frame False {
              # "dBc"
              n162 = local read "Fund"() -> (w317:ext)
            }
            frame True {
              # "dBFS"
            }
          }
          "Fund (compensated)" <- w285
          n163 = Subtract(x=w292, y=w290) -> (x-y=→"Window comp (dB)":dbl)
          n164 = local read "Amplitude Compensation"() -> (w306:ext)
          n165 = local read "Harmonic Spectrum"() -> (w299:ext[])
          n166 = local read "Sum of Harms 2"() -> (w296:ext)
          n167 = local read "Sum of Noise 2"() -> (w295:ext)
          n168 = local read "max Harmonic"() -> (w315:ext)
          n169 = Select(t=w306, s=FALSE, f=1.0) -> (s? t:f=w304:ext)
          n170 = local read "Sum of Noise"() -> (w316:ext)
          n171 = local read "Sum of Harms"() -> (w298:ext)
          n172 = Index Array(array=w299, index=3) -> (element=w300:ext)
          n173 = Index Array(array=w299, index=2) -> (element=w301:ext)
          n174 = Index Array(array=w299, index=0) -> (element=w312:ext)
          n175 = Index Array(array=w299, index=1) -> (element=w311:ext)
          n176 = formula code="SNRD=10*log(Fund*Gain/(SumNoise+SumHarm));\nSNR=10*log(Fund*Gain/SumNoise);\nTHD=10*log(Fund/SumHarm);\nSFDR=10*log(Fund/maxHarm);\nHarm2=10*log(Fund/H2);\nHarm3=10*log(Fund/H3);\nHarm4=10*log(Fund/H4);\nHarm5=10*log(Fund/H5);\nTHD2=10*log(Fund/SumHarm2);\nSNR2=10*log(Fund*Gain/SumNoise2);"("Fund"=w285, "SumNoise"=w316, "Gain"=w304, "maxHarm"=w315, "SumHarm"=w298, "H2"=w312, "H3"=w311, "H4"=w301, "H5"=w300, "SumHarm2"=w296, "SumNoise2"=w295) -> ("SNRD"=w269:dbl, "SNR"=→"SNR":dbl, "THD"=w270:dbl, "SFDR"=w271:dbl, "Harm2"=w272:dbl, "Harm3"=w273:dbl, "Harm4"=w274:dbl, "Harm5"=w275:dbl, "THD2"=w276:dbl, "SNR2"=w277:dbl)
          "SNRD" <- w269
          "THD (dBc)" <- w270
          "SFDR (dBc)" <- w271
          "2nd HD (dBc)" <- w272
          "3rd HD" <- w273
          "4th HD" <- w274
          "5th HD" <- w275
          "THD (dBc)" <- w276
          "SNR 2" <- w277
          n177 = Select(t="(dBFS)", s=w263, f="(dBc)") -> (s? t:f=w280:string)
          n178 = Concatenate Strings("SNRD ", w280) -> (w283:string)
          n179 = property on="SNRD" class="DigNum (strict)"("Caption.Text"=w283) -> ()  [unwired: 2 in, 2 out]
          n180 = Subtract(x=w269, y=w310) -> (x-y=w309:dbl)
          n181 = Subtract(x=w277, y=w310) -> (x-y=w308:dbl)
          n182 = Concatenate Strings("SNR ", w280) -> (w279:string)
          n183 = Divide(x=w309, y=w307) -> (x/y=w268:dbl)
          "ENOB" <- w268
          n184 = Divide(x=w308, y=w307) -> (x/y=w267:dbl)
          "enob" <- w267
          n185 = property on="SNR (dBFS)" class="Arr (strict)"("Caption.Text"=w279) -> ()  [unwired: 2 in, 2 out]
          n186 = property on="SNR 2" class="DigNum (strict)"("Caption.Text"=w279) -> ()  [unwired: 2 in, 2 out]
          n187 = local read "Ampl."() -> (w266:dbl)
          n188 = Build Array(w277, w271, w272, w273, w269, w276, w274, w275, w268, w267, w266) -> (→"Performance Array":dbl[])
        }
        frame #5 {
          w330 = ext[][] [[0.0, 0.1], [0.1, 0.2], [0.2, 0.30000000000000000001], [0.30000000000000000001, 0.4], [0.4, 0.5], [0.0, 0.5]]  # Frequency Bands (x FS)
          n189 = Unbundle By Name(w321) -> ("LoFreq (Hz)"=w320:ext, "HiFreq (Hz)"=w319:ext)
          n190 = local read "Actual Sampling Rate"() -> (w326:dbl)
          n191 = Build Array(w320, w319) -> (w327:ext[])
          n192 = Divide(x=w326, y=ext 1.0) -> (x/y=w324:ext)
          n193 = Divide(x=w327, y=w324) -> (x/y=w328:ext[])
          n194 = Build Array (concatenate)(w330, w328) -> (w329:ext[][])
          n195 = local read "Nyquist"() -> (w339:i32)
          n196 = local read "Actual Sampling Rate"() -> (w337:dbl)
          n197 = Multiply(x="BandMultiplier", y=w329) -> (x*y=w332:ext[][])
          n198 = Multiply(x=w339, y=2) -> (x*y=w336:i32)
          n199 = Multiply(x=w332, y=w336) -> (x*y=w346:ext[][])
          n200 = Divide(x=w337, y=w336) -> (x/y=w334:dbl)
          n201 = To Long Integer(number=w346) -> (32bit integer=w335:i32[][])
          n202 = Array Size(array=w332) -> (size(s)=w345:i32[])
          n203 = local read "Power Spec\n(No DC, Fund, Harmonics)"() -> (w342:ext[])
          n204 = Multiply(x=w335, y=w334) -> (x*y=w333:dbl[][])
          n205 = Index Array(array=w345, index=0) -> (element=w343:i32)
          n206 = Divide(x=w333, y=ext 1.0) -> (x/y=w322:ext[][])
          "Freq (Hz)" <- w322
          n207 = for {
            N: w343 -> [_]
            tunnel: w335 -> [w359] mode=indexing
            tunnel: w342 -> [w354]
            tunnel: [w352] -> w341 mode=indexing
            tunnel: [w348] -> w323 mode=indexing
            # "10*log10"
            n208 = Index Array(array=w359, index=1) -> (element=w358:i32)
            n209 = Index Array(array=w359, index=0) -> (element=w357:i32)
            n210 = Subtract(x=w358, y=w357) -> (x-y=w356:i32)
            n211 = local read "Fund (compensated)"() -> (w347:ext)
            n212 = Increment(x=w356) -> (x+1=w355:i32)
            n213 = Array Subset(array=w354, index=w357, length=w355) -> (w353:ext[])
            n214 = Add Array Elements(numeric array=w353) -> (sum=w352:ext)
            n215 = Divide(x=w347, y=w352) -> (x/y=w349:ext)
            n216 = Logarithm Base 10(1:w349) -> (0:w351:ext)
            n217 = Multiply(x=10.0, y=w351) -> (x*y=w348:ext)
          }
          "Noise Floor" <- w341
          "SNR (dBFS)" <- w323
        }
      }
    }
  }
  n218 = local read "PSRR/CMRR/BW"() -> (w20:T2)
  n219 = Bundle By Name(cluster=w20, "Fund(dB)"=w16, "SNR (dBFS)"=w3, "Freq (Hz)"=w2) -> (→"PSRR/CMRR/BW":T2)
  n220 = local read "ACParameter"() -> (w19:T3)
  n221 = Bundle By Name(cluster=w19, "ENOB"=w6, "enob"=w5, "SNRD(dB)"=w7, "THD (dBc)"=w8, "SFDR(dBc)"=w9, "2nd HD (dBc)"=w10, "3rd HD (dBc)"=w11, "4th HD (dBc)"=w12, "5th HD (dBc)"=w13, "THD (dBc)"=w14, "SNR(dBFS)"=w15, "WoSpur(dbFS)"=w17, "Ampl."=w4) -> (→"ACParameter":T3)
